vi "Display_LookUpGameRGB.vi"(1 "ActiveTile":T1, 4 "TilePixelOffset":i16) -> (15 "Red":bool, 16 "Green":bool, 17 "Blue":bool)   [LabVIEW 2018]
uses:
  TypDefs/Tile_Enum.ctl
  <vilib>/rvi/DataTransferAndStorage/Container/Common/niFpgaContainerExecOnDevCompGetState.vi
  <vilib>/rvi/Emulation/niFpgaEmulationIsFPGAContextNoSignature.vi
  <vilib>/rvi/DataTransferAndStorage/Container/Common/niFpgaContainerGetUniqueNameForEmu.vi
  <vilib>/rvi/Emulation/niFpgaProcessEmulError.vi
  <vilib>/rvi/Emulation/niFpgaSctlEmulationGetInTimedLoop.vi
  <vilib>/rvi/errors/nirviReportUnexpectedCaseInternalError (U32).vi
  <vilib>/rvi/Memory/Memory_Emulation/niFpgaMemoryEmulationCacheClearOnFirstRun.vi
  <vilib>/rvi/Memory/Memory_Emulation/nirvimemoryEmulationManagerCache_MakeExclusive.vi
  <vilib>/rvi/Memory/Memory_Emulation/niFpgaMemoryEmulationValidateCache.vi
  <vilib>/rvi/Memory/Memory_Emulation/nirvimemoryEmulationManagerCache_InsertValue.vi
  <vilib>/Utility/error.llb/Clear Errors.vi
  <vilib>/rvi/Memory/Memory_Emulation/nirvimemoryEmulationManagerCache_ReleaseExclusive.vi
  <vilib>/rvi/Memory/Memory_Emulation/nirvimemoryEmulationManagerCache_GetValue.vi
  <vilib>/rvi/Memory/Memory_Emulation/nirvimemoryEmulationManagerCache_SetValue.vi
  <vilib>/rvi/Emulation/niFpgaSctlEmulationResourceMgr.vi
  <vilib>/rvi/DataTransferAndStorage/Container/XNode/niFpgaContainer.xnode
  <vilib>/rvi/Memory/Memory_Emulation/niFpgaMemoryEmulationRefIn.vi
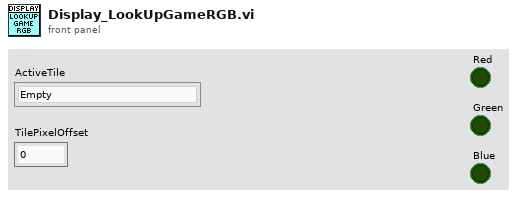
[diagram p1: front panel]
types:
  T1 = typedef "Tile_Enum.ctl" = enum8{"Empty", "Snake1_HeadPointingUp", "Snake1_HeadPointingDown", "Snake1_HeadPointingLeft", "Snake1_HeadPointingRight", "Snake1_DeadPointingUp", "Snake1_DeadPointingDown", "Snake1_DeadPointingLeft", "Snake1_DeadPointingRight", "Snake1_TailPointingUp", "Snake1_TailPointingDown", "Snake1_TailPointingLeft", "Snake1_TailPointingRight", "Snake1_Horizontal", "Snake1_Vertical", "Snake1_UpperLeftCorner", "Snake1_UpperRightCorner", "Snake1_LowerLeftCorner", "Snake1_LowerRightCorner", "Snake2_HeadPointingUp", "Snake2_HeadPointingDown", "Snake2_HeadPointingLeft", "Snake2_HeadPointingRight", "Snake2_DeadPointingUp", "Snake2_DeadPointingDown", "Snake2_DeadPointingLeft", "Snake2_DeadPointingRight", "Snake2_TailPointingUp", "Snake2_TailPointingDown", "Snake2_TailPointingLeft", "Snake2_TailPointingRight", "Snake2_Horizontal", "Snake2_Vertical", "Snake2_UpperLeftCorner", "Snake2_UpperRightCorner", "Snake2_LowerLeftCorner", "Snake2_LowerRightCorner", "Wall_Horizontal", "Wall_Vertical", "Wall_UpperLeftCorner", "Wall_UpperRightCorner", "Wall_LowerLeftCorner", "Wall_LowerRightCorner", "Pickup_SpeedUp", "Pickup_SlowDown", "Pickup_Banana", "Pickup_Grapes", "Pickup_Apple"}
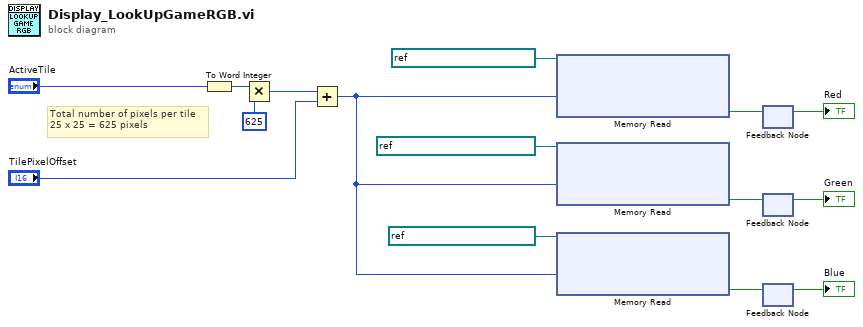
[diagram p0: block diagram]
diagram:
  # "Total number of pixels per tile\n25 x 25 = 625 pixels"
  n1 = To Word Integer(number="ActiveTile") -> (16bit integer=w9:i16)
  n2 = Multiply(x=w9, y=i16 625) -> (x*y=w10:i16)
  n3 = Add(x=w10, y="TilePixelOffset") -> (x+y=w8:i16)
  n4 = xnode ("Memory Read")("Address"=w8, "Memory In"=refnum<k21> "BlockMem_TilesetRed") -> ("Data"=w6:bool)  [unwired: 1 out]
  n5 = xnode ("Memory Read")("Address"=w8, "Memory In"=refnum<k21> "BlockMem_TilesetGreen") -> ("Data"=w5:bool)  [unwired: 1 out]
  n6 = xnode ("Memory Read")("Address"=w8, "Memory In"=refnum<k21> "BlockMem_TilesetBlue") -> ("Data"=w2:bool)  [unwired: 1 out]
  n7 = feedback #1() -> (→"Red":bool)  [unwired: 1 in]
  n8 = feedback-in #1(w6) -> ()
  n9 = feedback #2() -> (→"Green":bool)  [unwired: 1 in]
  n10 = feedback-in #2(w5) -> ()
  n11 = feedback #3() -> (→"Blue":bool)  [unwired: 1 in]
  n12 = feedback-in #3(w2) -> ()
